vi "BRig_dataExp_CueSwitch_PostR.vi"() -> (2 "output_CueSwitch_PostR":i32)   [LabVIEW 2014]
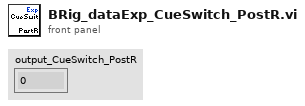
[diagram p1: front panel]
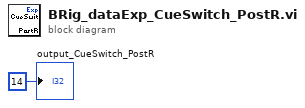
[diagram p0: block diagram]
diagram:
  "output_CueSwitch_PostR" <- 14 ("output_iBlock")
